vi "Get Event DVR.vi"(11 "Event Actor in":refnum<class "Event Actor.lvclass">) -> (2 "Event Self":map{string, refnum<data-value>}(c390))   [LabVIEW 2021, in "Event Actor.lvclass"]
uses:
  Event Actor.lvclass
  Msg/Msg.lvclass
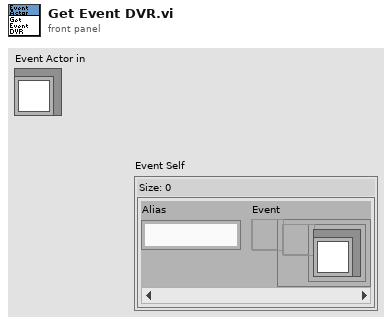
[diagram p1: front panel]
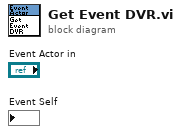
[diagram p0: block diagram]
diagram:
